vi "Constants.vi"() -> ()   [LabVIEW 2019, in "Inline Telemetry Prototype Shared.lvlib"]
doc: "Use this Global VI to access the GUIDs assigned to the page resources of the Custom Device."
uses:
  Inline Telemetry Prototype Shared.lvlib
panel:
  in  "Tab Control":enum32{"GUIDs", "Constants", "Properties"}(tab)
  in  "Page2":string="b525b825-7091-4b38-86e0-9ef956193000"
  in  "Page1":string="95400eec-0c66-4556-a185-e062850e8345"
  in  "Inline Telemetry Prototype":string="bb272428-986a-483c-8d4a-ae31e16c574f"
  in  "Compiled.Settings":string="Compiled.Settings"
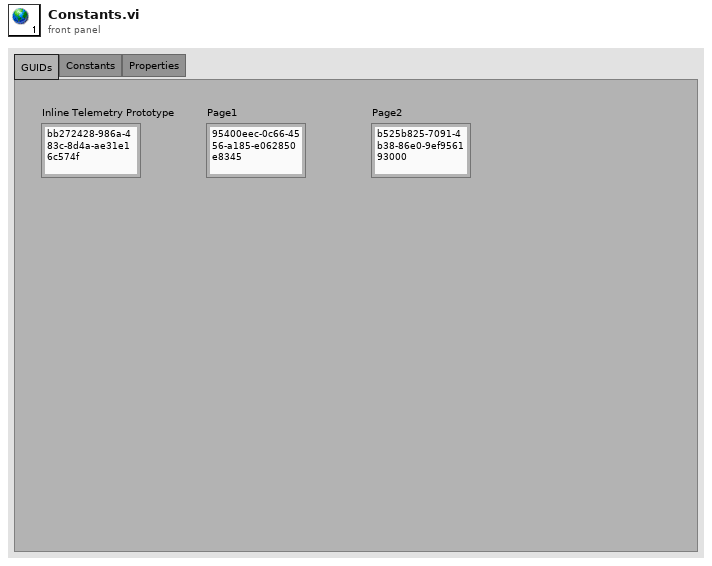
[diagram p1: front panel]
diagram:
